vi "Custom - Resize Pic and String.vi"(0 "m.width":i32, 1 "2D Picture":refnum<vi>, 2 "message ref":refnum<vi>, 5 "m.height":i32, 7 "p.width":i32, 9 "p.height":i32, 11 "error in (no error)":errorcluster, 12 "Message Location":enum16{"Top", "Bottom", "Right", "Left"}(ring)) -> (8 "Panel Width":i32, 10 "Panel Height":i32, 15 "error out":errorcluster)   [LabVIEW 2021, in "Pop-Up.lvlib" / "Popup.lvclass"]
doc: "update the sizing of the button and the image based on the calculated inputs and with padding\n\n<b>Code Developed By:</b> +\nDaniel Coons +\nhttps://github.com/danielcoons/tsc-pop-up"
uses:
  Popup.lvclass
  <vilib>/Utility/miscctls.llb/LVBoundsTypeDef.ctl
  <vilib>/Utility/miscctls.llb/LVPositionTypeDef.ctl
  <vilib>/Utility/miscctls.llb/LVPointTypeDef.ctl
  Popup.lvclass/Popup.ctl
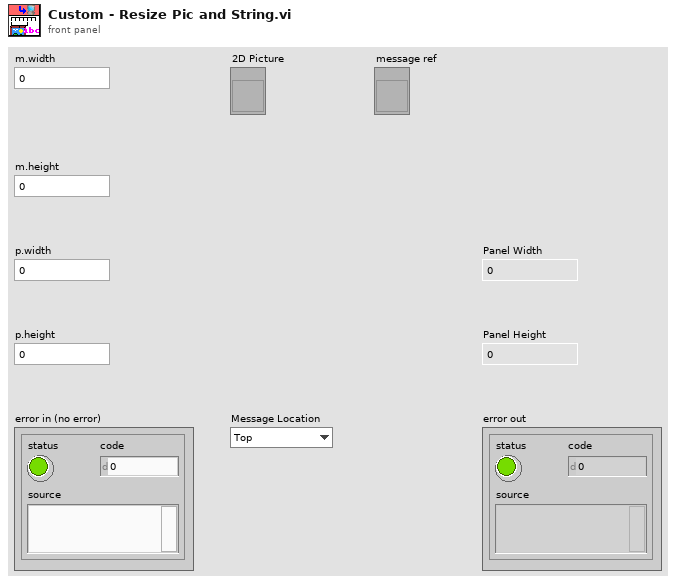
[diagram p1: front panel]
types:
  T1 = typedef "LVPointTypeDef.ctl" = cluster{"Horizontal":i16, "Vertical":i16}
  T2 = typedef "LVPositionTypeDef.ctl" = cluster{"Left":i32, "Top":i32}
  T3 = typedef "LVBoundsTypeDef.ctl" = cluster{"Width":u32, "Height":u32}
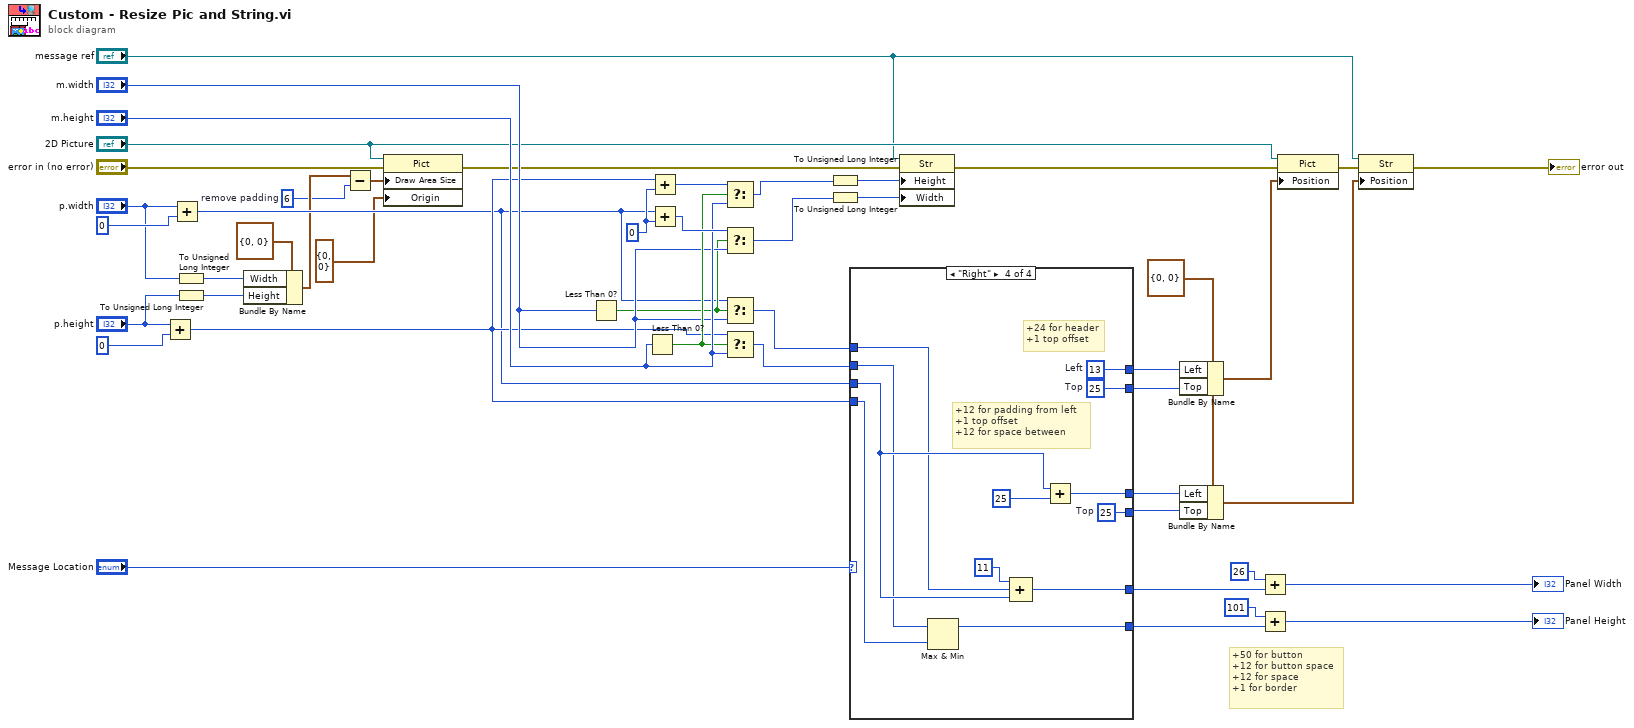
[diagram p0: block diagram]
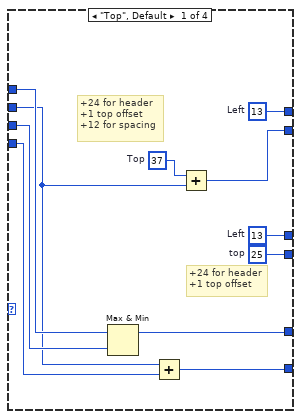
[diagram p2: hidden frame]
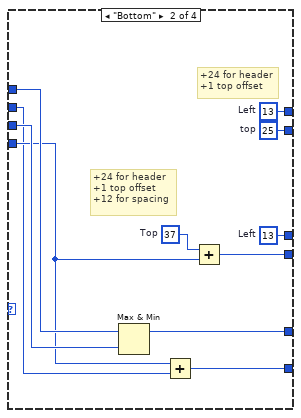
[diagram p3: hidden frame]
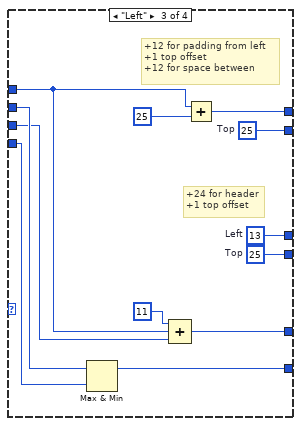
[diagram p4: hidden frame]
diagram:
  w8 = u32 6  # remove padding
  w15 = T2 {"Left"=0, "Top"=0} ("Position")
  w45 = 0 ("y")
  # "+50 for button\n+12 for button space\n+12 for space\n+1 for border"
  n1 = Add(x="p.height", y=0 ("x")) -> (x+y=w28:i32)
  n2 = Add(x="p.width", y=0 ("x")) -> (x+y=w26:i32)
  n3 = To Unsigned Long Integer(number="p.width") -> (unsigned 32bit integer=w36:u32)
  n4 = To Unsigned Long Integer(number="p.height") -> (unsigned 32bit integer=w37:u32)
  n5 = Bundle By Name(cluster=T3 {"Width"=0, "Height"=0} ("Draw Area Size"), "Width"=w36, "Height"=w37) -> (w20:T3)
  n6 = Subtract(x=w20, y=w8) -> (x-y=w9:T3)
  n7 = property class="Pict"(reference="2D Picture", error in="error in (no error)", "Draw Area Size"=w9, "Origin"=T1 {"Horizontal"=0, "Vertical"=0}) -> (error out=w24:errorcluster)  [unwired: 1 out]
  n8 = Less Than 0?(x="m.width") -> (x < 0?=w39:bool)
  n9 = Less Than 0?(x="m.height") -> (x < 0?=w42:bool)
  n10 = Add(x=w28, y=w45) -> (x+y=w46:i32)
  n11 = Add(x=w26, y=w45) -> (x+y=w44:i32)
  n12 = Select(t=w46, s=w42, f="m.height") -> (s? t:f=w47:i32)
  n13 = Select(t=w44, s=w39, f="m.width") -> (s? t:f=w41:i32)
  n14 = Select(t=w26, s=w39, f="m.width") -> (s? t:f=w38:i32)
  n15 = Select(t=w28, s=w42, f="m.height") -> (s? t:f=w32:i32)
  n16 = To Unsigned Long Integer(number=w47) -> (unsigned 32bit integer=w30:u32)
  n17 = To Unsigned Long Integer(number=w41) -> (unsigned 32bit integer=w31:u32)
  n18 = case shown="\"Right\"" "Message Location" {
    tunnel: [w57 w69 w72 w91] -> w19
    tunnel: [w56 w62 w73 w92] -> w18
    tunnel: [w55 w67 w76 w90] -> w17
    tunnel: [w54 w61 w75 w93] -> w16
    tunnel: w32 -> [w49 w59 w80 w85]
    tunnel: w38 -> [w51 w66 w70 w87]
    tunnel: w26 -> [w50 w65 w71 w88]
    tunnel: w28 -> [w48 w60 w79 w84]
    tunnel: [w53 w64 w81 w86] -> w33
    tunnel: [w52 w63 w78 w83] -> w34
    frame "Top", Default {
      w54 = 25  # top
      w58 = 37  # Top
      w55 = 13  # Left
      w57 = 13  # Left
      # "+24 for header\n+1 top offset"
      # "+24 for header\n+1 top offset\n+12 for spacing"
      n19 = Max & Min(x=w51, y=w50) -> (max(x,y)=w53:i32)  [unwired: 1 out]
      n20 = Add(x=w49, y=w48) -> (x+y=w52:i32)
      n21 = Add(x=w58, y=w49) -> (x+y=w56:i32)
    }
    frame "Bottom" {
      w62 = 25  # top
      w68 = 37  # Top
      w67 = 13  # Left
      w69 = 13  # Left
      # "+24 for header\n+1 top offset\n+12 for spacing"
      # "+24 for header\n+1 top offset"
      n22 = Max & Min(x=w66, y=w65) -> (max(x,y)=w64:i32)  [unwired: 1 out]
      n23 = Add(x=w60, y=w59) -> (x+y=w63:i32)
      n24 = Add(x=w68, y=w60) -> (x+y=w61:i32)
    }
    frame "Left" {
      w73 = 25  # Top
      w76 = 13  # Left
      w75 = 25  # Top
      # "+12 for padding from left\n+1 top offset\n+12 for space between"
      # "+24 for header\n+1 top offset"
      n25 = Max & Min(x=w80, y=w79) -> (max(x,y)=w78:i32)  [unwired: 1 out]
      n26 = Compound Arithmetic op=ADD(11 ("value"), w70, w71) -> (w81:i32)
      n27 = Add(x=w70, y=25) -> (x+y=w72:i32)
    }
    frame "Right" {
      w91 = 13  # Left
      w92 = 25  # Top
      w93 = 25  # Top
      # "+24 for header\n+1 top offset"
      # "+12 for padding from left\n+1 top offset\n+12 for space between"
      n28 = Max & Min(x=w85, y=w84) -> (max(x,y)=w83:i32)  [unwired: 1 out]
      n29 = Compound Arithmetic op=ADD(11 ("value"), w87, w88) -> (w86:i32)
      n30 = Add(x=w88, y=25) -> (x+y=w90:i32)
    }
  }
  n31 = property class="Str"(reference="message ref", error in=w24, "Height"=w30, "Width"=w31) -> (error out=w7:errorcluster)  [unwired: 1 out]
  n32 = Bundle By Name(cluster=w15, "Left"=w19, "Top"=w18) -> (w5:T2)
  n33 = Bundle By Name(cluster=w15, "Left"=w17, "Top"=w16) -> (w2:T2)
  n34 = Add(x=26, y=w33) -> (x+y=→"Panel Width":i32)
  n35 = Add(x=101, y=w34) -> (x+y=→"Panel Height":i32)
  n36 = property class="Pict"(reference="2D Picture", error in=w7, "Position"=w5) -> (error out=w4:errorcluster)  [unwired: 1 out]
  n37 = property class="Str"(reference="message ref", error in=w4, "Position"=w2) -> (error out=→"error out":errorcluster)  [unwired: 1 out]
